vi "FL Get Membership Function.vi"   [LabVIEW 2013, in "NI_Fuzzy_Logic_API.lvlib"]
doc: "Returns the shape, color, and points of a membership function for a linguistic variable. You can return a membership function from a fuzzy system or from an array of membership functions. The data type you wire to the <B>fuzzy system in</B> input determines the polymorphic instance to use."
uses:
  <vilib>/addons/Fuzzy Logic/NI_Fuzzy_Logic_API.lvlib
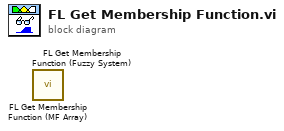
[diagram p0: block diagram]
diagram:
  n1 = call <vilib>:"FL Get Membership Function (MF Array).vi"() -> ()  [unwired: 9 in, 7 out]
  n2 = call <vilib>:"FL Get Membership Function (Fuzzy System).vi"() -> ()  [unwired: 9 in, 7 out]
